vi "set_template_file.vi"(8 "error in (no error)":errorcluster, 10 "Path":path, 11 "Boc12 in":refnum<class "Boc12.lvclass">) -> (0 "error out":errorcluster, 3 "Boc12 out":refnum<class "Boc12.lvclass">)   [LabVIEW 2017, in "Boc12.lvclass"]
uses:
  Boc12.lvclass
  Report.lvclass/Report.ctl
  Report.lvclass
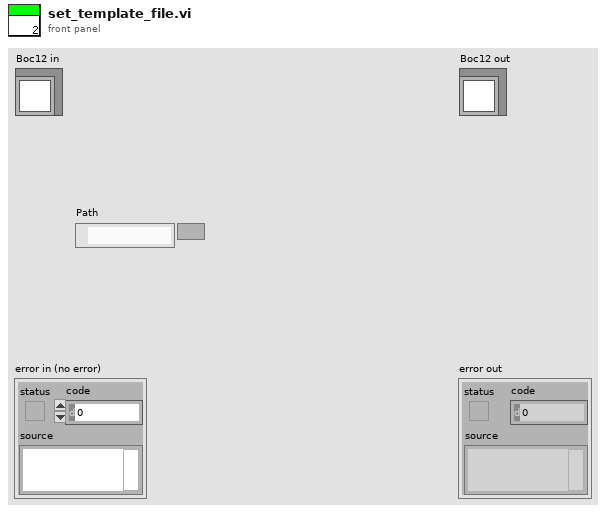
[diagram p1: front panel]
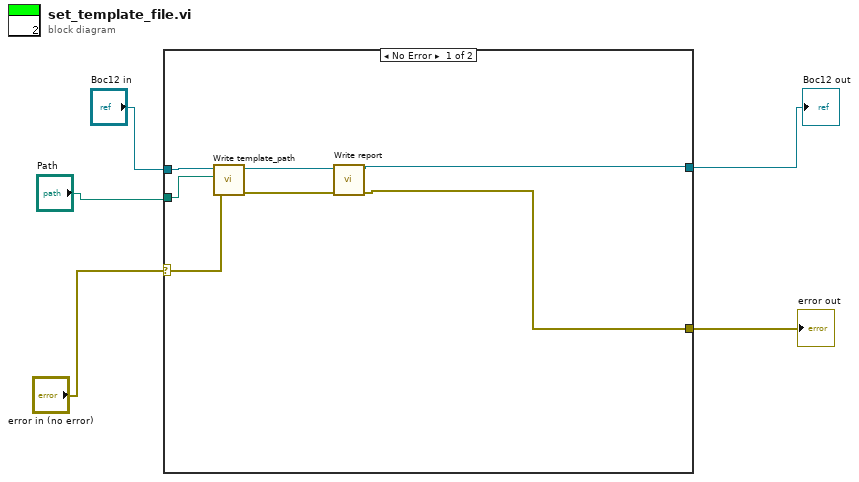
[diagram p0: block diagram]
diagram:
  n1 = case shown="No Error" "error in (no error)" {
    selector: "error in (no error)" -> [w10 w13]
    tunnel: "Boc12 in" -> [w12 w14]
    tunnel: "Path" -> [w11 _]
    tunnel: [w7 w14] -> w2
    tunnel: [w6 w13] -> w1
    frame No Error {
      n2 = call "Write template_path.vi"("error in (no error)"=w10, "template_path"=w11, "Report in"=w12) -> ("error out"=w8:errorcluster, "Report out"=w9:refnum<class "Boc12.lvclass">)  [unwired: 7 in]
      n3 = call-dynamic "Write report.vi"("error in (no error)"=w8, "Boc12 in"=w9) -> ("error out"=w6:errorcluster, "Boc12 out"=w7:refnum<class "Boc12.lvclass">)  [unwired: 8 in]
    }
    frame Error {
    }
  }
  "error out" <- w1
  "Boc12 out" <- w2
